vi "Report Error to Main.vi"(7 "clear error (T)":bool=TRUE, 10 "error in (no error)":errorcluster, 11 "subpanel to main command event":T1) -> (2 "error out":errorcluster, 3 "reported error?":bool)   [LabVIEW 2017, in "NI_Robotics_Configure Steering Frame.lvlib"]
uses:
  <vilib>/robotics/Dialog/Configure Steering Frame/NI_Robotics_Configure Steering Frame.lvlib
  <vilib>/robotics/Dialog/Configure Steering Frame/Subpanel to Main Command Event.ctl
  <vilib>/robotics/Dialog/Configure Steering Frame/Subpanel to Main Command.ctl
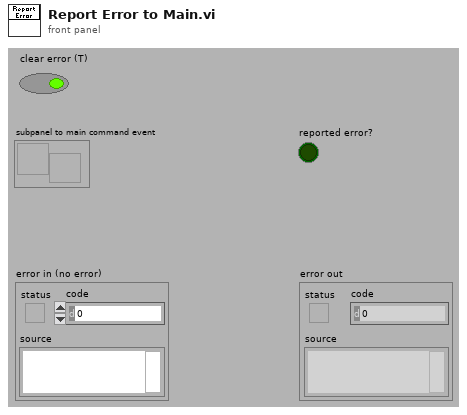
[diagram p1: front panel]
types:
  T1 = typedef "NI_Robotics_Configure Steering Frame.lvlib/Subpanel to Main Command Event.ctl" = refnum<user-event>
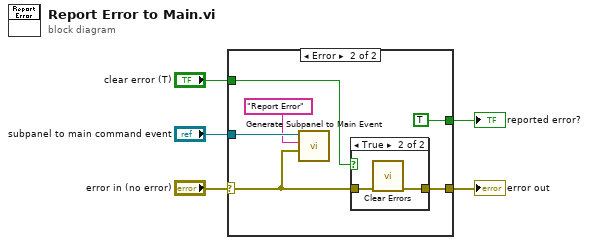
[diagram p0: block diagram]
diagram:
  n1 = case shown="Error" "error in (no error)" {
    selector: "error in (no error)" -> [w6 w8]
    tunnel: [w6 w7] -> w4
    tunnel: "subpanel to main command event" -> [_ w12]
    tunnel: [_ TRUE] -> w2
    tunnel: "clear error (T)" -> [_ w9]
    frame No Error {
    }
    frame Error {
      n2 = call <vilib>:"Generate Subpanel to Main Event.vi"("data"=w8, "command"="Report Error", "subpanel to main command event"=w12) -> ()  [unwired: 8 in, 1 out]
      n3 = case shown="True" w9 {
        tunnel: w8 -> [w13 w15]
        tunnel: [w13 w14] -> w7
        frame False {
        }
        frame True {
          n4 = call <vilib>:"Clear Errors.vi"("error in (no error)"=w15) -> ("error out"=w14:errorcluster)  [unwired: 5 in, 1 out]
        }
      }
    }
  }
  "error out" <- w4
  "reported error?" <- w2
